vi "Frame.Export.vi"(8 "error in (no error)":errorcluster, 11 "Item Ref in":T1 format="%.0x") -> (0 "error out":errorcluster, 2 "Frame":T2 {"Signals"."Byte Order" items=["Little Endian", "Big Endian"]; "Signals"."Data Type" items=["Signed", "Unsigned", "IEEE Float"]}, 3 "Item Ref out":T1 format="%.0x")   [LabVIEW 2024, in "Diagnostics Addon System Explorer.lvlib"]
uses:
  Diagnostics Addon System Explorer.lvlib
  Types/Frame.Export.ctl
  Addon Shared/Types/Signal.ctl
  <vilib>/NI VeriStand/Custom Device API/Custom Device Item Ref.ctl
  Types/FG.Action.ctl
  Signal.FG.vi
  Frame.GetSignalRefs.vi
  Addon Shared/SubVIs/Constants.vi
  <vilib>/NI/NI VeriStand Advanced SysDef API/SysDef API/SysDef.Property.Set.vi
  <vilib>/NI/NI VeriStand Advanced SysDef API/_SubVIs/SysDef.Property.Set.U32.vi
  <vilib>/NI VeriStand/Custom Device API/NI VeriStand - Get Item Property.vi
  <vilib>/NI VeriStand/Custom Device API/Get Item Property (U32).vi
  <vilib>/NI VeriStand/Custom Device Tools/Custom Device Utility Library/NI VeriStand - Search for Item.vi
  <vilib>/NI VeriStand/Custom Device Tools/Custom Device Utility Library/NI VeriStand - Search for Item by GUID.vi
  <vilib>/NI VeriStand/Custom Device API/NI VeriStand - Get Item Children.vi
  <vilib>/NI/NI VeriStand Advanced SysDef API/_SubVIs/SysDef.Property.Set.DBL.vi
  <vilib>/NI/NI VeriStand Advanced SysDef API/_SubVIs/SysDef.Property.Set.String.vi
  <vilib>/NI VeriStand/Custom Device API/Get Item Property (Double).vi
  <vilib>/NI VeriStand/Custom Device API/Get Item Property (String).vi
  <vilib>/NI VeriStand/Custom Device API/NI VeriStand - Get Custom Device Channel Data.vi
  <vilib>/NI VeriStand/Custom Device API/Custom Device API.lvlib
  Addon Shared/Diagnostics Addon Shared.lvlib
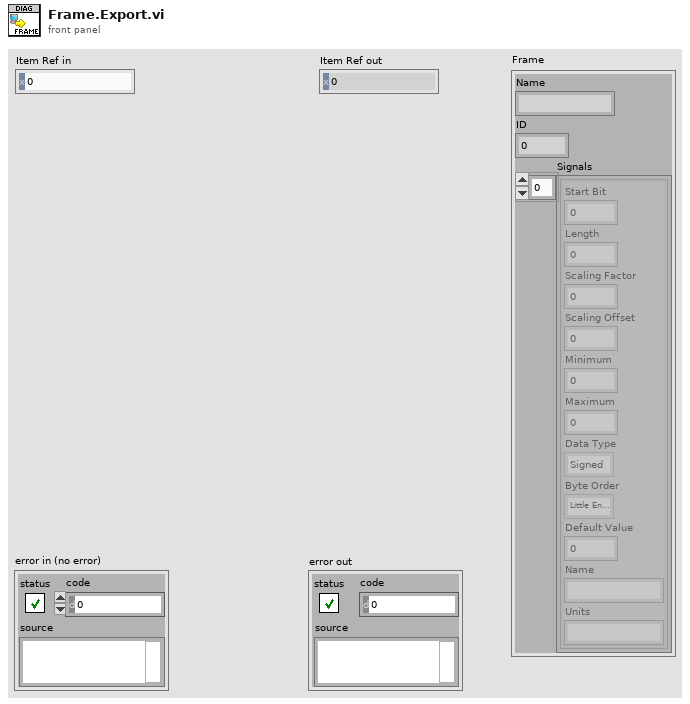
[diagram p1: front panel]
types:
  T1 = typedef "Custom Device API.lvlib/Custom Device Item Ref.ctl" = u64
  T2 = typedef "Diagnostics Addon System Explorer.lvlib/Frame.Export.ctl" = cluster{"Name":string, "ID":u32, "Signals":T3[]}
  T3 = typedef "Diagnostics Addon Shared.lvlib/Signal.ctl" = cluster{"Start Bit":u32, "Length":u32, "Scaling Factor":dbl, "Scaling Offset":dbl, "Minimum":dbl, "Maximum":dbl, "Data Type":u32, "Byte Order":u32, "Default Value":dbl, "Name":string, "Units":string}
  T4 = typedef "Diagnostics Addon System Explorer.lvlib/FG.Action.ctl" = enum16{"Get", "Set"}
  T5 = typedef "Custom Device API.lvlib/Custom Device Item Info.ctl" = cluster{"Name":string, "Is Channel":bool, "GUID":string, "Is Waveform":bool}
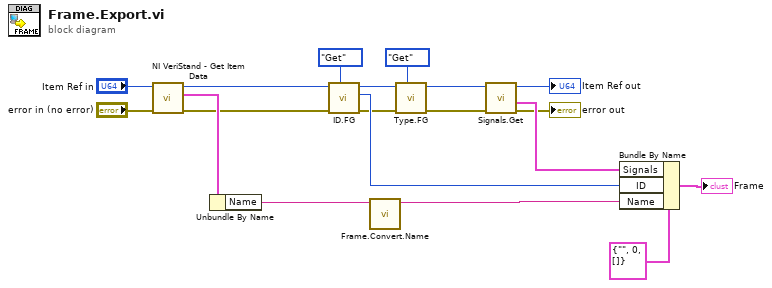
[diagram p0: block diagram]
diagram:
  n1 = call <vilib>:"NI VeriStand - Get Item Data.vi"("error in (no error)"="error in (no error)", "Item Ref in"="Item Ref in") -> ("error out"=w2:errorcluster, "Item Info"=w19:T5, "Item Ref out"=w1:T1)  [unwired: 7 out]
  n2 = Unbundle By Name(w19) -> ("Name"=w4:string)
  n3 = call "ID.FG.vi"("Action"=FG.Action."Get", "error in (no error)"=w2, "Device Item Ref in"=w1) -> ("error out"=w7:errorcluster, "ID"=w16:u32, "Device Item Ref out"=w18:T1)  [unwired: 6 in]
  n4 = call "Frame.Convert.Name.vi"("VS Frame Name"=w4) -> ("Frame Name"=w3:string)  [unwired: 9 in, 1 out]
  n5 = call "Type.FG.vi"("Action"=FG.Action."Get", "error in (no error)"=w7, "Device Item Ref in"=w18) -> ("error out"=w6:errorcluster, "Device Item Ref out"=w8:T1)  [unwired: 6 in, 1 out]
  n6 = call "Signals.Get.vi"("error in (no error)"=w6, "Device Item Ref out"=w8) -> ("error out"=→"error out":errorcluster, "Parameters"=w15:T3[], "Item Ref out"=→"Item Ref out":T1)  [unwired: 6 in, 1 out]
  n7 = Bundle By Name(cluster=T2 {"Name"="", "ID"=0, "Signals"=[]} ("PID In"), "Signals"=w15, "ID"=w16, "Name"=w3) -> (→"Frame":T2)
